vi "Fehlermeldungen (SubVI).vi"(0 "Fehler 1":bool, 1 "Fehler 2":bool, 2 "Fehler 3":bool, 3 "Fehler 4":bool, 4 "Fehler 5":bool, 5 "Fehler 6":bool, 6 "Fehler 7":bool, 7 "Fehler 8":bool, 8 "Fehlermeldungen Namen":string, 9 "Fehler 9":bool, 10 "Kritischefehler Positionen":string, 11 "Fehler 10":bool) -> (20 "Fehlermeldung Ausgang":string="Zeit ist größer als Zykluslänge", 21 "Fehler?":bool, 22 "Sperre":bool)   [LabVIEW 2010]
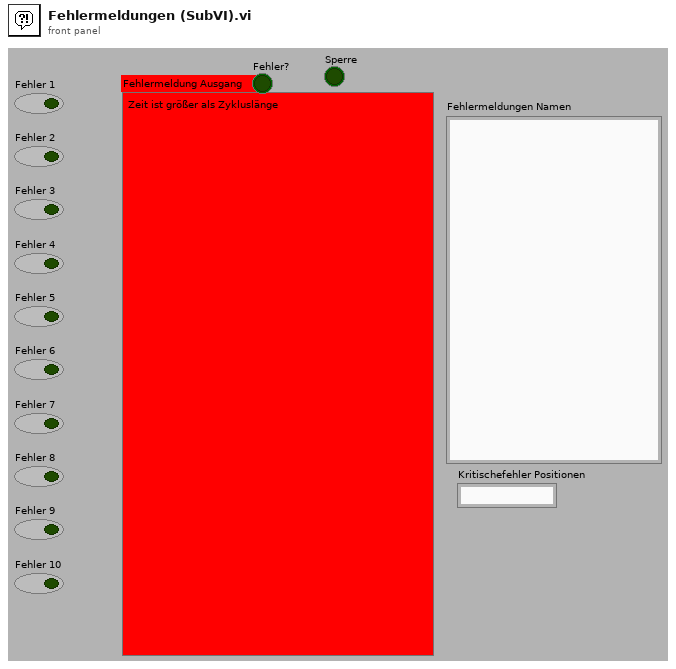
[diagram p1: front panel]
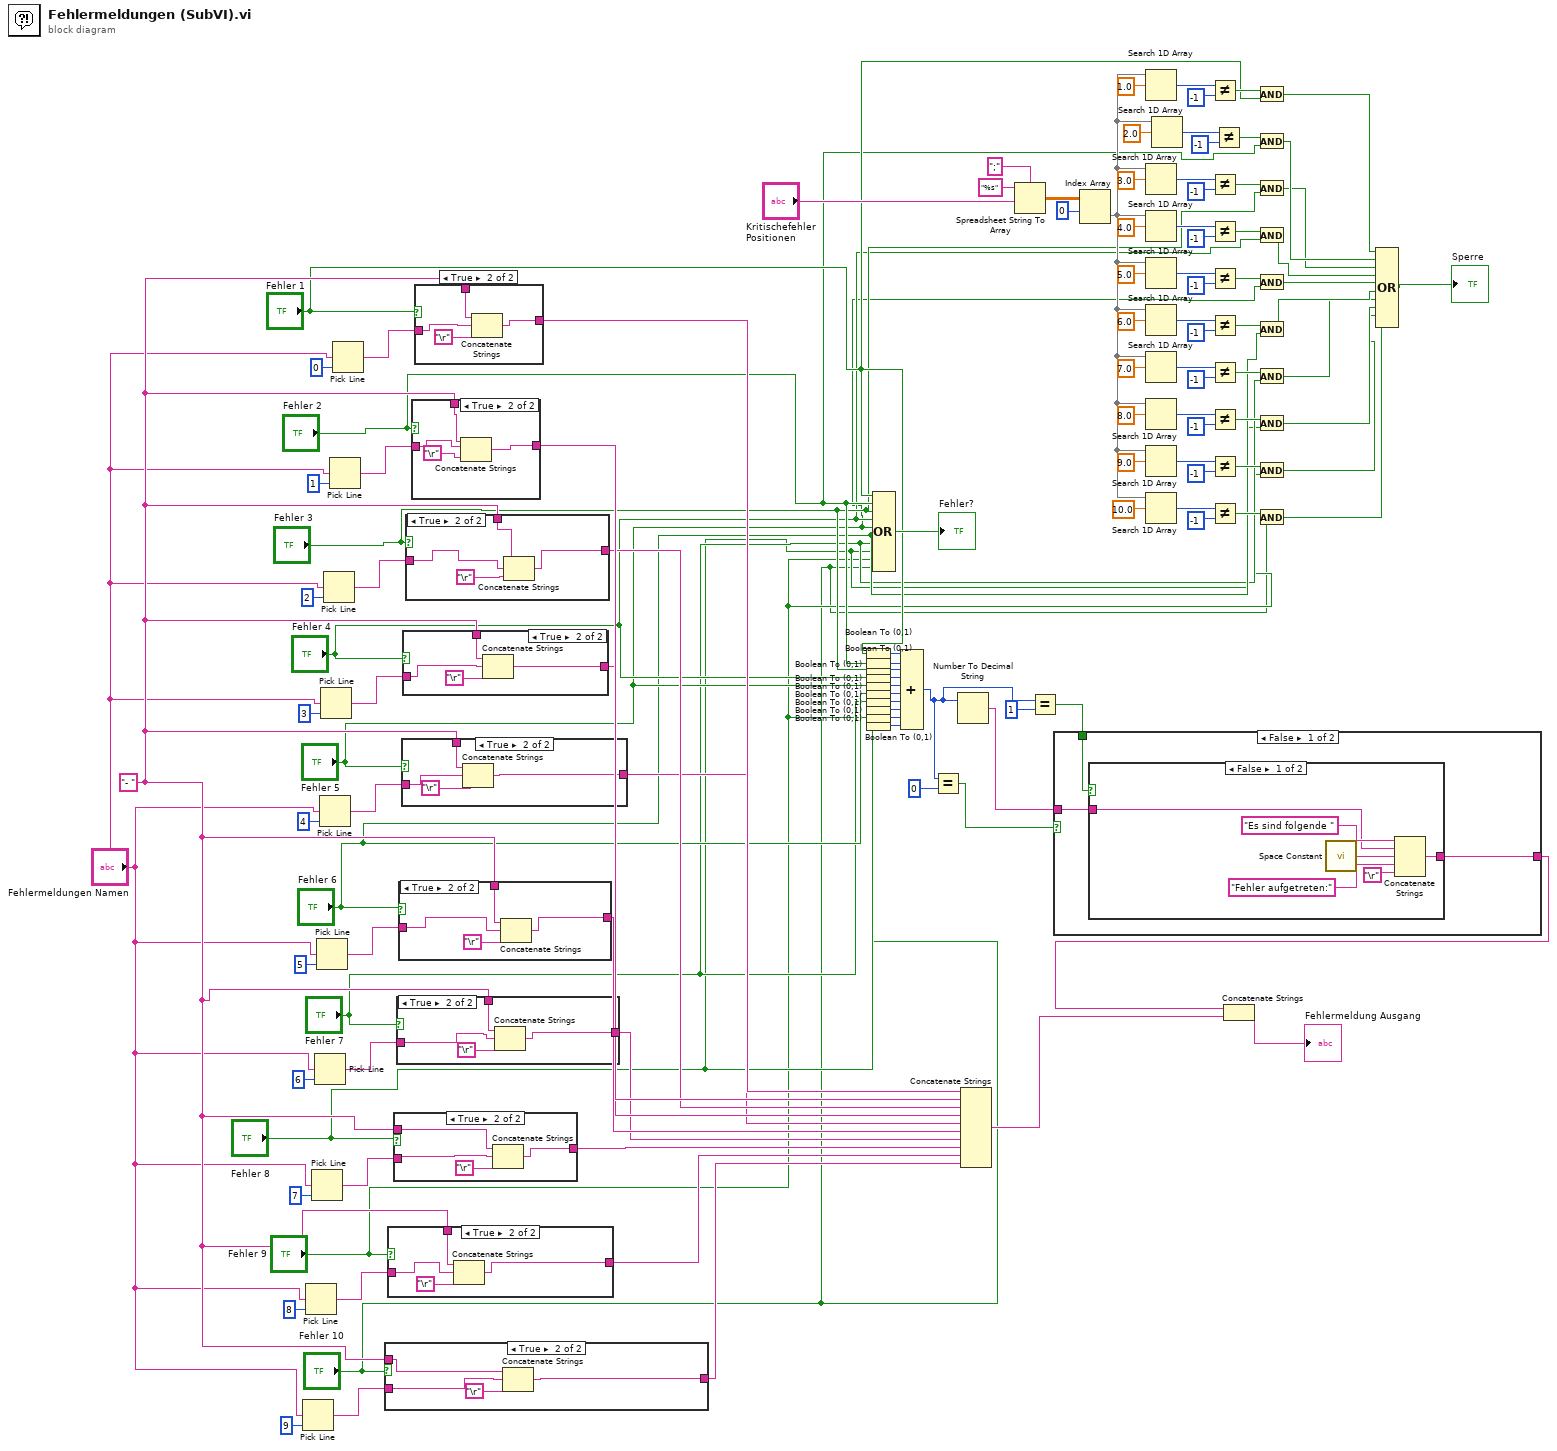
[diagram p0: block diagram]
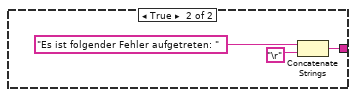
[diagram p2: hidden frame]
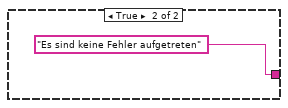
[diagram p3: hidden frame]
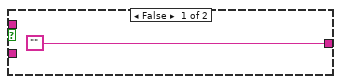
[diagram p4: hidden frame]
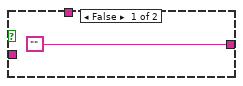
[diagram p5: hidden frame]
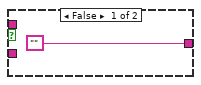
[diagram p6: hidden frame]
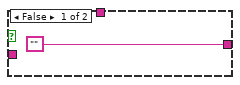
[diagram p7: hidden frame]
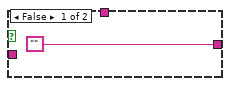
[diagram p8: hidden frame]
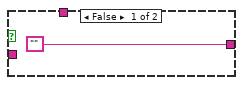
[diagram p9: hidden frame]
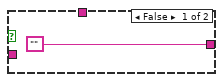
[diagram p10: hidden frame]
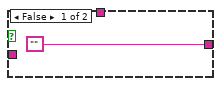
[diagram p11: hidden frame]
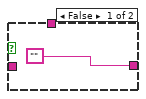
[diagram p12: hidden frame]
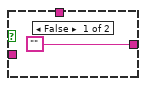
[diagram p13: hidden frame]
diagram:
  w71 = "- " ("String")
  n1 = Pick Line(multi-line string="Fehlermeldungen Namen", line index=9 ("Zeilenindex")) -> (output string=w100:string)  [unwired: 1 in]
  n2 = Pick Line(multi-line string="Fehlermeldungen Namen", line index=8 ("Zeilenindex")) -> (output string=w102:string)  [unwired: 1 in]
  n3 = Pick Line(multi-line string="Fehlermeldungen Namen", line index=7 ("Zeilenindex")) -> (output string=w104:string)  [unwired: 1 in]
  n4 = Pick Line(multi-line string="Fehlermeldungen Namen", line index=6 ("Zeilenindex")) -> (output string=w106:string)  [unwired: 1 in]
  n5 = Pick Line(multi-line string="Fehlermeldungen Namen", line index=5 ("Zeilenindex")) -> (output string=w108:string)  [unwired: 1 in]
  n6 = Pick Line(multi-line string="Fehlermeldungen Namen", line index=4 ("Zeilenindex")) -> (output string=w110:string)  [unwired: 1 in]
  n7 = Pick Line(multi-line string="Fehlermeldungen Namen", line index=3 ("Zeilenindex")) -> (output string=w112:string)  [unwired: 1 in]
  n8 = Pick Line(multi-line string="Fehlermeldungen Namen", line index=2 ("Zeilenindex")) -> (output string=w114:string)  [unwired: 1 in]
  n9 = Pick Line(multi-line string="Fehlermeldungen Namen", line index=1 ("Zeilenindex")) -> (output string=w116:string)  [unwired: 1 in]
  n10 = Pick Line(multi-line string="Fehlermeldungen Namen", line index=0 ("Zeilenindex")) -> (output string=w118:string)  [unwired: 1 in]
  n11 = case shown="True" "Fehler 10" {
    tunnel: ["" w123] -> w90
    tunnel: w100 -> [_ w121]
    tunnel: w71 -> [_ w122]
    frame False {
    }
    frame True {
      n12 = Concatenate Strings(w122, w121, "\r") -> (w123:string)
    }
  }
  n13 = case shown="True" "Fehler 9" {
    tunnel: ["" w128] -> w91
    tunnel: w102 -> [_ w126]
    tunnel: w71 -> [_ w127]
    frame False {
    }
    frame True {
      n14 = Concatenate Strings(w127, w126, "\r") -> (w128:string)
    }
  }
  n15 = case shown="True" "Fehler 8" {
    tunnel: ["" w133] -> w92
    tunnel: w104 -> [_ w131]
    tunnel: w71 -> [_ w132]
    frame False {
    }
    frame True {
      n16 = Concatenate Strings(w132, w131, "\r") -> (w133:string)
    }
  }
  n17 = case shown="True" "Fehler 7" {
    tunnel: ["" w138] -> w93
    tunnel: w106 -> [_ w136]
    tunnel: w71 -> [_ w137]
    frame False {
    }
    frame True {
      n18 = Concatenate Strings(w137, w136, "\r") -> (w138:string)
    }
  }
  n19 = case shown="True" "Fehler 6" {
    tunnel: ["" w143] -> w94
    tunnel: w108 -> [_ w141]
    tunnel: w71 -> [_ w142]
    frame False {
    }
    frame True {
      n20 = Concatenate Strings(w142, w141, "\r") -> (w143:string)
    }
  }
  n21 = case shown="True" "Fehler 5" {
    tunnel: ["" w148] -> w95
    tunnel: w110 -> [_ w147]
    tunnel: w71 -> [_ w146]
    frame False {
    }
    frame True {
      n22 = Concatenate Strings(w146, w147, "\r") -> (w148:string)
    }
  }
  n23 = case shown="True" "Fehler 4" {
    tunnel: ["" w153] -> w96
    tunnel: w112 -> [_ w152]
    tunnel: w71 -> [_ w151]
    frame False {
    }
    frame True {
      n24 = Concatenate Strings(w151, w152, "\r") -> (w153:string)
    }
  }
  n25 = case shown="True" "Fehler 3" {
    tunnel: ["" w158] -> w97
    tunnel: w114 -> [_ w157]
    tunnel: w71 -> [_ w156]
    frame False {
    }
    frame True {
      n26 = Concatenate Strings(w156, w157, "\r") -> (w158:string)
    }
  }
  n27 = case shown="True" "Fehler 2" {
    tunnel: w116 -> [_ w162]
    tunnel: ["" w164] -> w98
    tunnel: w71 -> [_ w161]
    frame False {
    }
    frame True {
      n28 = Concatenate Strings(w161, w162, "\r") -> (w164:string)
    }
  }
  n29 = case shown="True" "Fehler 1" {
    tunnel: ["" w168] -> w99
    tunnel: w118 -> [_ w167]
    tunnel: w71 -> [_ w166]
    frame False {
    }
    frame True {
      n30 = Concatenate Strings(w166, w167, "\r") -> (w168:string)
    }
  }
  n31 = Boolean To (0,1)(Boolean="Fehler 1") -> (0, 1=w89:i16)
  n32 = Boolean To (0,1)(Boolean="Fehler 2") -> (0, 1=w88:i16)
  n33 = Boolean To (0,1)(Boolean="Fehler 3") -> (0, 1=w87:i16)
  n34 = Boolean To (0,1)(Boolean="Fehler 4") -> (0, 1=w86:i16)
  n35 = Boolean To (0,1)(Boolean="Fehler 5") -> (0, 1=w85:i16)
  n36 = Boolean To (0,1)(Boolean="Fehler 6") -> (0, 1=w84:i16)
  n37 = Boolean To (0,1)(Boolean="Fehler 7") -> (0, 1=w83:i16)
  n38 = Boolean To (0,1)(Boolean="Fehler 8") -> (0, 1=w82:i16)
  n39 = Boolean To (0,1)(Boolean="Fehler 9") -> (0, 1=w81:i16)
  n40 = Boolean To (0,1)(Boolean="Fehler 10") -> (0, 1=w80:i16)
  n41 = Compound Arithmetic op=OR("Fehler 1", "Fehler 2", "Fehler 3", "Fehler 4", "Fehler 5", "Fehler 6", "Fehler 7", "Fehler 8", "Fehler 9", "Fehler 10") -> (→"Fehler?":bool)
  n42 = Compound Arithmetic op=ADD(w89, w88, w87, w86, w85, w84, w83, w82, w81, w80) -> (w75:i16)
  n43 = Equal?(x=w75, y=i16 0) -> (x = y?=w74:bool)
  n44 = Number To Decimal String(number=w75) -> (decimal integer string=w77:string)  [unwired: 1 in]
  n45 = Concatenate Strings(w99, w98, w97, w96, w95, w94, w93, w92, w91, w90) -> (w70:string)
  n46 = Spreadsheet String To Array(delimiter (Tab)=";" ("Trennzeichen (Tabulator)"), format string="%s" ("Format-String"), spreadsheet string="Kritischefehler Positionen") -> (array=w65:dbl[][])  [unwired: 1 in]
  n47 = Equal?(x=w75, y=i16 1) -> (x = y?=w78:bool)
  n48 = case shown="False" w74 {
    tunnel: w78 -> [w172 _]
    tunnel: [w171 "Es sind keine Fehler aufgetreten"] -> w73
    tunnel: w77 -> [w170 _]
    frame False {
      n49 = case shown="False" w172 {
        tunnel: [w174 w179] -> w171
        tunnel: w170 -> [w173 _]
        frame False {
          n50 = call <vilib>:"Space Constant.vi"() -> ("String"=w177:string)
          n51 = Concatenate Strings("Es sind folgende ", w173, w177, "Fehler aufgetreten:", "\r") -> (w174:string)
        }
        frame True {
          n52 = Concatenate Strings("Es ist folgender Fehler aufgetreten: ", "\r") -> (w179:string)
        }
      }
    }
    frame True {
    }
  }
  n53 = Index Array(array=w65, index (row)=0 ("Index (Zeile)")) -> (element=w53:dbl[])  [unwired: 1 in]
  n54 = Search 1D Array(1D array=w53, element=1.0 ("Element")) -> (index of element=w41:i32)  [unwired: 1 in]
  n55 = Search 1D Array(1D array=w53, element=3.0 ("Element")) -> (index of element=w38:i32)  [unwired: 1 in]
  n56 = Search 1D Array(1D array=w53, element=4.0 ("Element")) -> (index of element=w37:i32)  [unwired: 1 in]
  n57 = Search 1D Array(1D array=w53, element=5.0 ("Element")) -> (index of element=w36:i32)  [unwired: 1 in]
  n58 = Search 1D Array(1D array=w53, element=6.0 ("Element")) -> (index of element=w35:i32)  [unwired: 1 in]
  n59 = Search 1D Array(1D array=w53, element=7.0 ("Element")) -> (index of element=w34:i32)  [unwired: 1 in]
  n60 = Search 1D Array(1D array=w53, element=8.0 ("Element")) -> (index of element=w33:i32)  [unwired: 1 in]
  n61 = Search 1D Array(1D array=w53, element=9.0 ("Element")) -> (index of element=w39:i32)  [unwired: 1 in]
  n62 = Search 1D Array(1D array=w53, element=10.0 ("Element")) -> (index of element=w40:i32)  [unwired: 1 in]
  n63 = Search 1D Array(1D array=w53, element=2.0 ("Element")) -> (index of element=w42:i32)  [unwired: 1 in]
  n64 = Not Equal?(x=w41, y=-1) -> (x != y?=w31:bool)
  n65 = Not Equal?(x=w38, y=-1) -> (x != y?=w28:bool)
  n66 = Not Equal?(x=w37, y=-1) -> (x != y?=w27:bool)
  n67 = Not Equal?(x=w36, y=-1) -> (x != y?=w26:bool)
  n68 = Not Equal?(x=w35, y=-1) -> (x != y?=w25:bool)
  n69 = Not Equal?(x=w34, y=-1) -> (x != y?=w24:bool)
  n70 = Not Equal?(x=w33, y=-1) -> (x != y?=w23:bool)
  n71 = Not Equal?(x=w39, y=-1) -> (x != y?=w22:bool)
  n72 = Not Equal?(x=w40, y=-1) -> (x != y?=w30:bool)
  n73 = Not Equal?(x=w42, y=-1) -> (x != y?=w29:bool)
  n74 = Concatenate Strings(w73, w70) -> (→"Fehlermeldung Ausgang":string)
  n75 = And(x=w31, y="Fehler 1") -> (x .and. y?=w11:bool)
  n76 = And(x=w29, y="Fehler 2") -> (x .and. y?=w10:bool)
  n77 = And(x=w28, y="Fehler 3") -> (x .and. y?=w9:bool)
  n78 = And(x=w27, y="Fehler 4") -> (x .and. y?=w8:bool)
  n79 = And(x=w26, y="Fehler 5") -> (x .and. y?=w7:bool)
  n80 = And(x=w25, y="Fehler 6") -> (x .and. y?=w6:bool)
  n81 = And(x=w24, y="Fehler 7") -> (x .and. y?=w5:bool)
  n82 = And(x=w23, y="Fehler 8") -> (x .and. y?=w4:bool)
  n83 = And(x=w22, y="Fehler 9") -> (x .and. y?=w3:bool)
  n84 = And(x=w30, y="Fehler 10") -> (x .and. y?=w2:bool)
  n85 = Compound Arithmetic op=OR(w11, w10, w9, w8, w7, w6, w5, w4, w3, w2) -> (→"Sperre":bool)
